vi "Unpack to 4-byte Packet Words.vi"(0 "serialized data in":u8[](array[numeric])=[0, 0, 0, 0, 0, 0, 0, 0], 1 "reset":bool, 5 "valid bytes in":fxp<+,4,4>, 9 "input valid":bool, 12 "ready for output":bool) -> (4 "serialized data out":u8[](array[numeric]), 6 "valid bytes out":fxp<+,3,3>, 10 "output valid":bool, 14 "ready for input":bool)   [LabVIEW 2020, in "GettingStarted_Acq_Tap_148X_FPGA.lvlib"]
uses:
  132812b1-2bbb-4e50-a4da-7e7653350c20.vi
  GettingStarted_Acq_Tap_148X_FPGA.lvlib
types:
  T1 = cluster{"serialized data in":u8[], "t":fxp<+,3,3>}
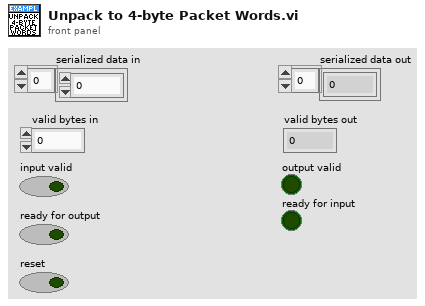
[diagram p1: front panel]
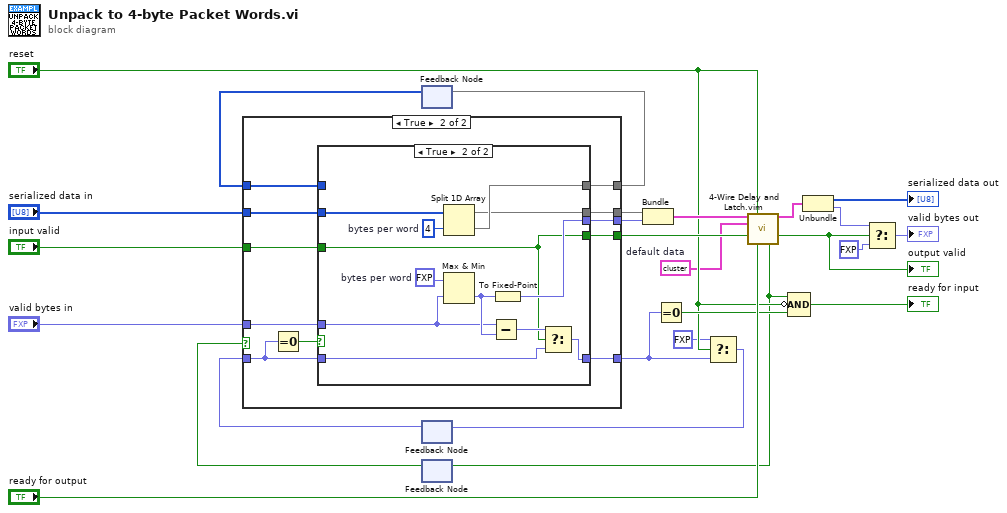
[diagram p0: block diagram]
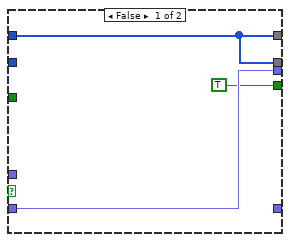
[diagram p3: hidden frame]
diagram:
  w1 = T1 {"serialized data in"=[0, 0, 0, 0], "t"=0.0}  # default data
  n1 = feedback #1() -> (w17:u8[])  [unwired: 1 in]
  n2 = feedback #2() -> (w19:fxp<+,3,3>)  [unwired: 1 in]
  n3 = feedback #3() -> (w22:bool)  [unwired: 1 in]
  n4 = case shown="True" w22 {
    tunnel: "serialized data in" -> [_ w32]
    tunnel: "valid bytes in" -> [_ w36]
    tunnel: [w28 w35] -> w4
    tunnel: w19 -> [w28 w38]
    tunnel: [_ w37] -> w16
    tunnel: [w27 w31] -> w18
    tunnel: w17 -> [w27 w34]
    tunnel: [w27 w33] -> w15
    tunnel: [_ w30] -> w10
    tunnel: "input valid" -> [_ w29]
    frame False {
    }
    frame True {
      n5 = Equal To 0?(x=w38) -> (x = 0?=w39:bool)
      n6 = case shown="True" w39 {
        tunnel: w38 -> [w42 w46]
        tunnel: [w42 w49] -> w37
        tunnel: w36 -> [_ w47]
        tunnel: [_ w44] -> w35
        tunnel: w34 -> [w41 _]
        tunnel: [w41 w52] -> w33
        tunnel: w32 -> [_ w54]
        tunnel: [w41 w53] -> w31
        tunnel: [TRUE w43] -> w30
        tunnel: w29 -> [_ w43]
        frame False {
        }
        frame True {
          w51 = 4  # bytes per word
          w50 = fxp<+,4,4> 4.0  # bytes per word
          n7 = Split 1D Array(array=w54, index=w51) -> (first subarray=w52:u8[], second subarray=w53:u8[])
          n8 = Max & Min(x=w50, y=w47) -> (min(x,y)=w48:fxp<+,4,4>)  [unwired: 1 out]
          n9 = Subtract(x=w47, y=w48) -> (x-y=w45:fxp<+,3,3>)
          n10 = To Fixed-Point(number=w48) -> (fixed-point=w49:fxp<+,3,3>)  [unwired: 1 in]
          n11 = Select(t=w45, s=w43, f=w46) -> (s? t:f=w44:fxp<+,3,3>)
        }
      }
    }
  }
  n12 = feedback-in #1(w18) -> ()
  n13 = Bundle("serialized data in"=w15, "t"=w16) -> (w14:T1)  [unwired: 1 in]
  n14 = Equal To 0?(x=w4) -> (x = 0?=w7:bool)
  n15 = Select(t=fxp<+,3,3> 0.0, s="reset", f=w4) -> (s? t:f=w3:fxp<+,3,3>)
  n16 = feedback-in #2(w3) -> ()
  n17 = call "4-Wire Delay and Latch.vim"("data in"=w14, "reset"="reset", "default data"=w1, "input valid"=w10, "ready for output"="ready for output") -> ("data out"=w13:T1, "output valid"=w24:bool, "ready for input"=w2:bool)  [unwired: 8 in]
  "output valid" <- w24
  n18 = feedback-in #3(w2) -> ()
  n19 = Compound Arithmetic op=AND(w2, invert "reset", w7) -> (→"ready for input":bool)
  n20 = Unbundle(w13) -> ("serialized data in"=→"serialized data out":u8[], "t"=w11:fxp<+,3,3>)
  n21 = Select(t=w11, s=w24, f=fxp<+,3,3> 0.0 ("valid bytes out")) -> (s? t:f=→"valid bytes out":fxp<+,3,3>)
